vi "add_ChannelFloat32_roslv.vi"(4 "ChannelFloat32":cluster{"name":string, "values":sgl[]}, 5 "msg in":string) -> (2 "msg out":string)   [LabVIEW 2014]
doc: "Flattens an float32 array into a message"
uses:
  std_msgs/subs/stringScalar_roslv.vi
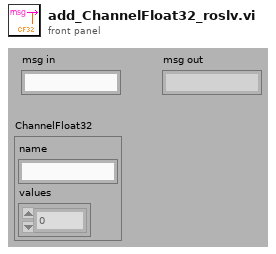
[diagram p1: front panel]
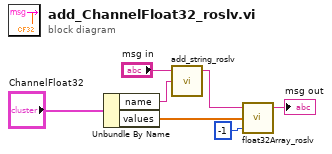
[diagram p0: block diagram]
diagram:
  n1 = Unbundle By Name("ChannelFloat32") -> ("name"=w2:string, "values"=w3:sgl[])
  n2 = call-poly "add_string_roslv.vi"("String"=w2, "msg in"="msg in") -> ("msg out"=w5:string)  [unwired: 3 in]
  n3 = call "float32Array_roslv.vi"("Array Length"=-1, "Array"=w3, "msg in"=w5) -> ("msg out"=→"msg out":string)  [unwired: 2 in]
